vi "test_simple_examples with timeout.vi"() -> ()   [LabVIEW 2018, in "LV-0mq-Julia_roundtrip-lib.lvlib"]
uses:
  LV-0mq-Julia_roundtrip-lib.lvlib
  Server or client state.ctl
  detailed error info.ctl
  StackFrame.ctl
  simple examples functions.ctl
  ZMQ timeouts.ctl
  Commands.ctl
  commands LV2Jl.ctl
  482f2ec0-5302-44bb-bdd2-45c372870067.vi
  edf81fa3-46bf-427f-9605-85b461656974.vi
  d2cb43a9-9305-42fb-ad58-bce983510195.vi
  9182218e-1e17-4e73-8c4b-7de0f475a335.vi
  35a44a82-786b-41ea-be73-9a4468e4df9d.vi
  482f2ec0-5302-44bb-bdd2-45c372870067.vi/9ed5a05b-029a-4cf9-8f74-86d17c033540.vi
  482f2ec0-5302-44bb-bdd2-45c372870067.vi/431fdeb3-535d-48a6-80d3-ce07043e4822.vi
  482f2ec0-5302-44bb-bdd2-45c372870067.vi/6e3a5974-e93f-4958-8e58-bfe5222df237.vi
  edf81fa3-46bf-427f-9605-85b461656974.vi/dd2a08ad-0639-467b-9435-389f4bd48a85.vi
  d2cb43a9-9305-42fb-ad58-bce983510195.vi/e28c4e1c-617d-4a26-8291-f58a5accd33d.vi
  d2cb43a9-9305-42fb-ad58-bce983510195.vi/697b26af-9cff-4296-98ec-fa9d12ca8fdc.vi
  d2cb43a9-9305-42fb-ad58-bce983510195.vi/17159f77-75f5-4b7b-8d47-844af2eb1bcd.vi
  9182218e-1e17-4e73-8c4b-7de0f475a335.vi/6b7feeb5-19de-417f-bcbc-aec3b1e8345f.vi
  9182218e-1e17-4e73-8c4b-7de0f475a335.vi/7970c5bc-6f8c-498d-9eee-822ea5f26e23.vi
  9182218e-1e17-4e73-8c4b-7de0f475a335.vi/2f2cc08c-6f15-46a0-b24a-2c0737e5dd5e.vi
  35a44a82-786b-41ea-be73-9a4468e4df9d.vi/edd291af-888e-4547-8763-33a9db2b2a61.vi
  35a44a82-786b-41ea-be73-9a4468e4df9d.vi/9c0ac3f0-dad9-4795-8f5f-702d875dafaa.vi
  edf81fa3-46bf-427f-9605-85b461656974.vi/dd2a08ad-0639-467b-9435-389f4bd48a85.vi/1040e0bc-00ab-48b1-9004-b2897991f2c6.vi
  35a44a82-786b-41ea-be73-9a4468e4df9d.vi/edd291af-888e-4547-8763-33a9db2b2a61.vi/c75629c6-22a1-4cf2-848a-1de687213dd2.vi
  35a44a82-786b-41ea-be73-9a4468e4df9d.vi/edd291af-888e-4547-8763-33a9db2b2a61.vi/58d0dd4f-d013-483e-a73a-a72c22b2f5d6.vi
  edf81fa3-46bf-427f-9605-85b461656974.vi/dd2a08ad-0639-467b-9435-389f4bd48a85.vi/1040e0bc-00ab-48b1-9004-b2897991f2c6.vi/e9506487-c1a2-4aa8-b83c-f353e91e5b82.vi
  35a44a82-786b-41ea-be73-9a4468e4df9d.vi/edd291af-888e-4547-8763-33a9db2b2a61.vi/c75629c6-22a1-4cf2-848a-1de687213dd2.vi/f86c6b3b-20ab-4607-a249-4edff951d1c3.vi
  check ID validity.vi
  bindata_descr to JSON.vi
  check cluster field names.vi
  concat JSON.vi
  <vilib>/Utility/error.llb/Error Cluster From Error Code.vi
  <vilib>/measure/NI_MABase.lvlib
panel:
  out "fns":string[](array[string])
  out "ZMQ prev Timeouts out":T1={"SNDTIMEO"=-1, "RCVTIMEO"=-1}
  out "Jl Server state":T2
  in  "execution control pages":enum32{"Start", "go - test"}(tab)
  in  "go":bool caption="go (Julia Server started externally)"
  in  "Start with Julia":bool caption="Start Julia Server and go"
  in  "p":dbl=1.0
  in  "fn":T3 caption="select function at Server" items=["arr_amplitude", "arr_length", "arr_mean", "arr_median", "arr_rms", "vec_amplify", "vec_attenuate", "vec_power"]
  in  "trim_at_begin":dbl
  in  "trim_at_end":dbl
  in  "Group":T4(tab)
  out "Server response":dbl
  out "data received plot":dbl[](graph)
  out "data received":dbl[](array[numeric]) format="%.3f"
  out "RMS":dbl
  out "detailed error info":T5
  out "current error":errorcluster
  out "final error":errorcluster
  out "short err code":u8
  in  "tones":T7(array[cluster])=[{"frequency"=10.0, "amplitude"=1.0, "phase"=0.0}, {"frequency"=20.0, "amplitude"=0.1, "phase"=0.0}] {"phase" format="%.2p"; "amplitude" format="%0.2p"; "frequency" format="%0.2p"}
  in  "noise (rms)":dbl=0.1 format="%.2p"
  in  "offset":dbl format="%.2p"
  in  "sampling info":cluster{"Fs":dbl, "#s":dbl}={"Fs"=1000.0, "#s"=1000.0} {"Fs" format="%.2p"}
  in  "next":bool
  out "data sent to server":dbl[](graph)
  out "data sent":dbl[](array[numeric]) format="%.3f"
  out "function name":string
  in  "stop this VI only":bool
  in  "stop both this VI and Julia Server":bool
  # "generate sample array"
  # "function and parameter"
  # "enter a negative or a large positive value to cause an exception"
  # "data returned by server"
  # "data sent to server"
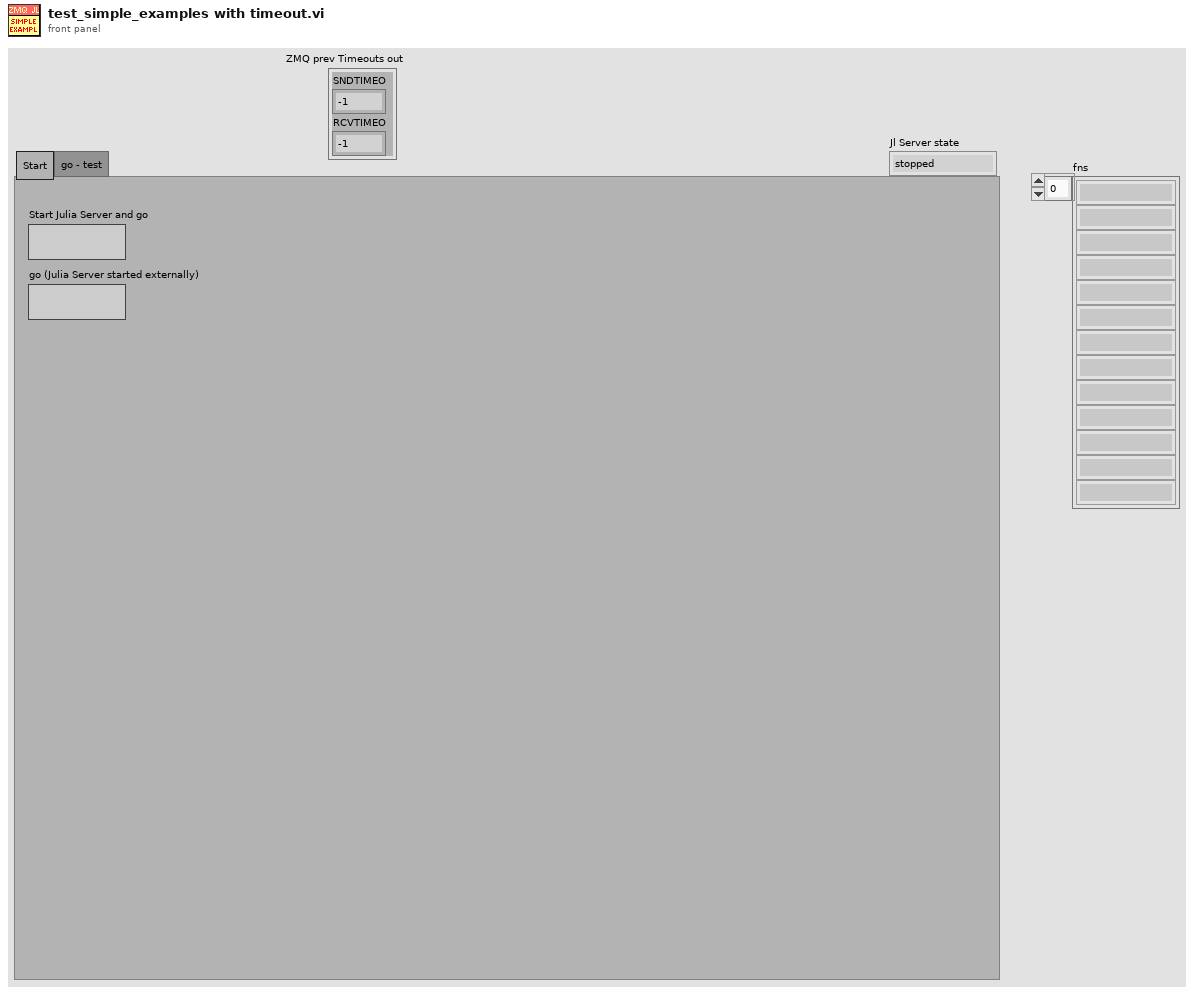
[diagram p1: front panel]
types:
  T1 = typedef "LV-0mq-Julia_roundtrip-lib.lvlib/ZMQ timeouts.ctl" = cluster{"SNDTIMEO":i32, "RCVTIMEO":i32}
  T2 = typedef "LV-0mq-Julia_roundtrip-lib.lvlib/Server or client state.ctl" = enum16{"stopped", "running", "unknown"}
  T3 = typedef "LV-0mq-Julia_roundtrip-lib.lvlib/simple examples functions.ctl" = u16
  T4 = enum32{"fns returning scalar", "fns returning vector", "error"}
  T5 = typedef "LV-0mq-Julia_roundtrip-lib.lvlib/detailed error info.ctl" = cluster{"exception_or_info":string, "trace":T6[]}
  T6 = typedef "LV-0mq-Julia_roundtrip-lib.lvlib/StackFrame.ctl" = cluster{"frame_summary":string, "func":string, "linfo":string, "file":string, "line":i32, "pointer":u64, "from_c":bool, "inlined":bool}
  T7 = cluster{"frequency":dbl, "amplitude":dbl, "phase":dbl}[]
  T8 = typedef "LV-0mq-Julia_roundtrip-lib.lvlib/commands LV2Jl.ctl" = u8
  T9 = typedef "LV-0mq-Julia_roundtrip-lib.lvlib/Commands.ctl" = enum16{"Start Jl-server & Init LV-client", "Send request & Get response ", "Stop Jl-server & Cleanup LV-client", "Cleanup LV-client", "Start Jl-server", "Stop Jl-server", "Init LV-Client", "Cleanup LV-Client", "(not allowed)", "Set LV Client state", "Set Jl Server state", "set ZMQ timeout", "read ZMQ timeout", "read-out state"}
  T10 = enum8{"Enabled", "Disabled", "Disabled and Grayed Out"}
  T11 = typedef "LV-0mq-Julia_roundtrip-lib.lvlib/Bindata&description.ctl" = cluster{"bindata_descr":T12[], "bindata":u8[]}
  T12 = typedef "LV-0mq-Julia_roundtrip-lib.lvlib/Bindata description.ctl" = cluster{"nofbytes":i32, "numtype":string, "start":i32, "arrdims":i32[], "kwarg_name":string, "category":string}
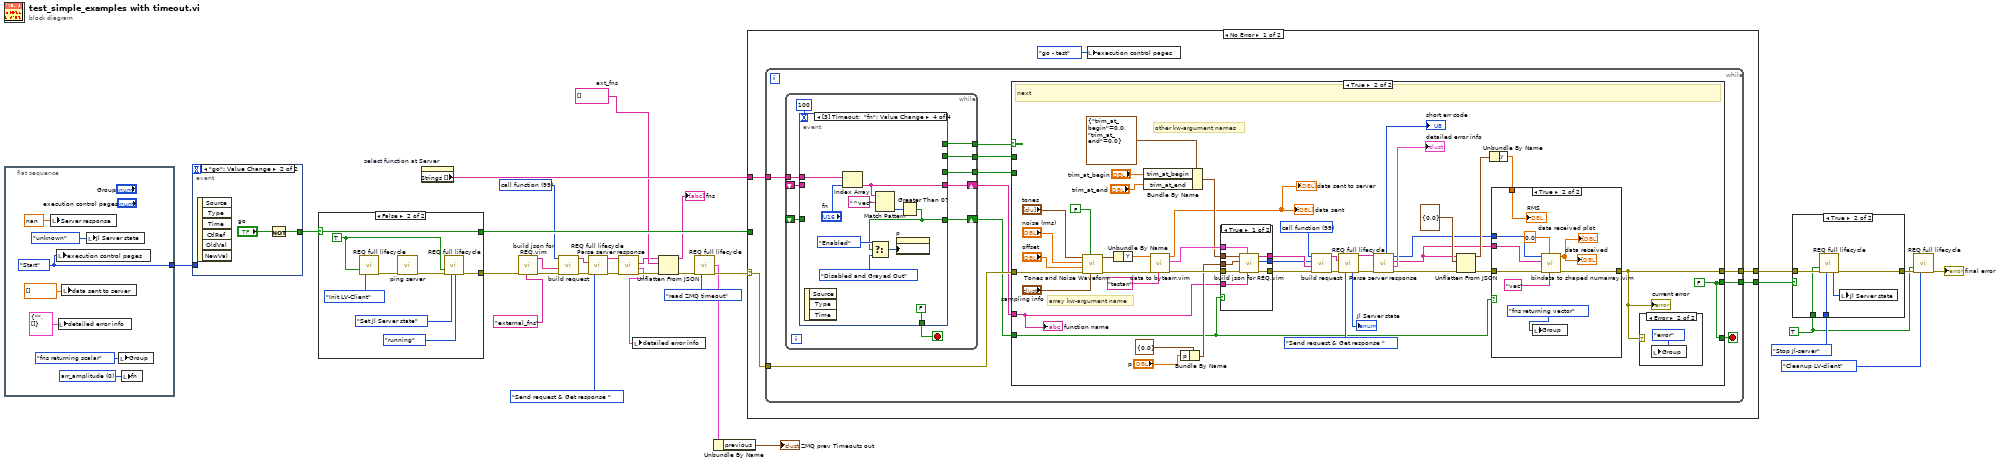
[diagram p0: block diagram]
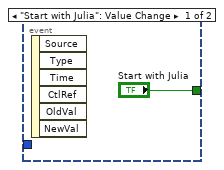
[diagram p2: hidden frame]
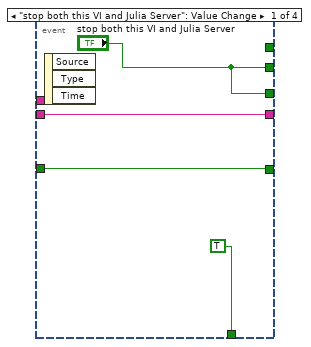
[diagram p3: hidden frame]
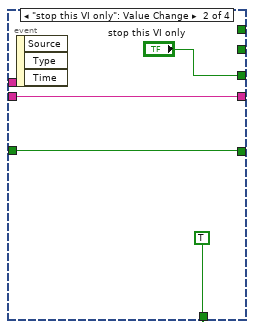
[diagram p4: hidden frame]
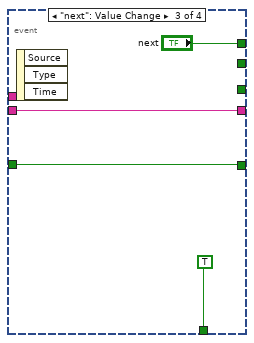
[diagram p5: hidden frame]
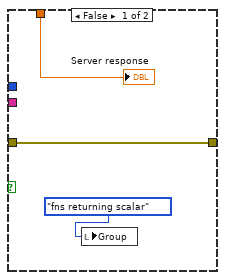
[diagram p7: hidden frame]
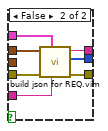
[diagram p8: hidden frame]
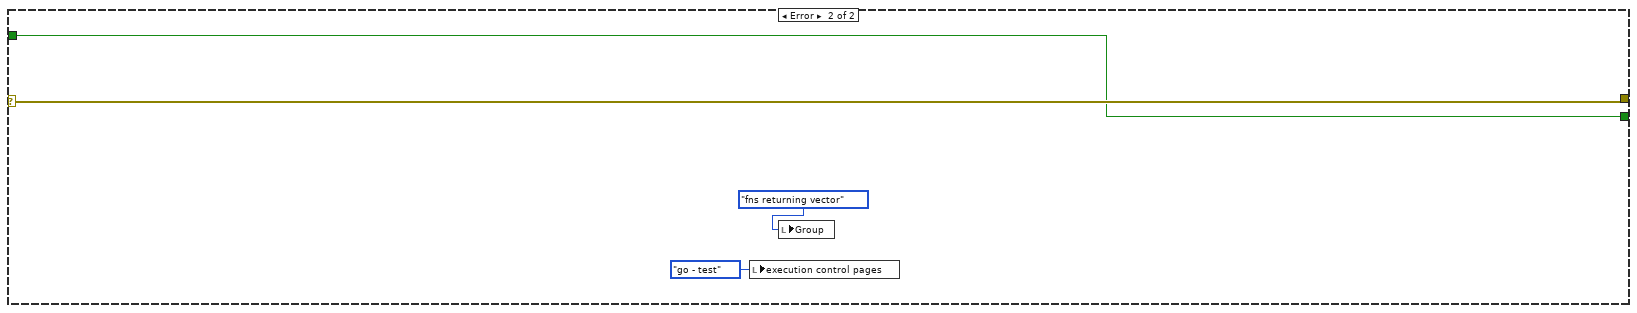
[diagram p10: hidden frame]
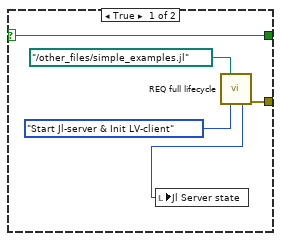
[diagram p11: hidden frame]
diagram:
  w4 = string[] []  # ext_fns
  w13 = T8 99 items=["call function"=99, "ping"=112, "stop"=115, "unused"=254] ("Command")
  w26 = TRUE ("Force command")
  n1 = flat-sequence {
    tunnel: [w38] -> w21
    frame #0 {
      w32 = T3 0 items=["arr_amplitude", "arr_length", "arr_mean", "arr_median", "arr_rms", "vec_amplify", "vec_attenuate", "vec_power"] ("fn")
      w38 = enum32{"Start", "go - test", "finish"}."Start" ("execution control pages")
      n2 = local write "Server response"(nan ("Server response")) -> ()
      n3 = local write "execution control pages"(w38) -> ()
      n4 = local write "detailed error info"(T5 {"exception_or_info"="", "trace"=[]} ("detailed error info")) -> ()
      n5 = local write "data sent to server"(dbl[] []) -> ()
      n6 = local write "Jl Server state"(Server_or_client_state."unknown" ("Jl Server state out")) -> ()
      n7 = local write "Group"(T4."fns returning scalar" ("Group")) -> ()
      n8 = local write "fn"(w32) -> ()
    }
  }
  n9 = event shown="[1] \"go\": Value Change" {
    selector: _ -> [_ _]
    dyn-events: _ -> [_ _]
    timeout: _ -> [_ _]
    tunnel: ["Start with Julia" w40] -> w24
    tunnel: w21 -> [_ _]
    event "Start with Julia": Value Change {
      n10 = event-data() -> ()  [unwired: 1 in, 6 out]
    }
    event "go": Value Change {
      n11 = event-data() -> ()  [unwired: 1 in, 6 out]
      n12 = Not(x="go") -> (.not. x?=w40:bool)
    }
  }
  n13 = case shown="False" w24 {
    selector: w24 -> [w43 w49]
    tunnel: [w45 w50] -> w12
    tunnel: [w43 w49] -> w22
    frame True {
      n14 = call "REQ full lifecycle.vi"("Julia user functions script"=path "../other_files/simple_examples.jl", "command"=Commands."Start Jl-server & Init LV-client") -> ("Jl Server state out"=w42:T2, "error out"=w45:errorcluster)  [unwired: 7 in, 5 out]
      n15 = local write "Jl Server state"(w42) -> ()
    }
    frame False {
      w52 = TRUE ("Force command")
      n16 = call "REQ full lifecycle.vi"("Force command"=w52, "command"=Commands."Init LV-Client") -> ("error out"=w48:errorcluster)  [unwired: 7 in, 6 out]
      n17 = call "ping server.vi"("error in"=w48) -> ("error out"=w47:errorcluster)  [unwired: 9 in, 1 out]
      n18 = call "REQ full lifecycle.vi"("Force command"=w52, "error in"=w47, "command"=Commands."Set Jl Server state", "Jl Server state in"=Server_or_client_state."running") -> ("error out"=w50:errorcluster)  [unwired: 5 in, 6 out]
    }
  }
  n19 = property on="select function at Server" class="Ring (strict)"() -> ("Strings []"=w23:string[])  [unwired: 2 in, 2 out]
  n20 = call "build json for REQ.vim"("fun2call"="external_fns", "error in (no error)"=w12) -> ("error out"=w11:errorcluster, "JSON string out"=w10:string)  [unwired: 7 in, 1 out]
  n21 = call "build request.vi"("error in (no error)"=w11, "JSON data"=w10, "Command"=w13) -> ("error out"=w15:errorcluster, "REQ string"=w14:string)  [unwired: 7 in]
  n22 = call "REQ full lifecycle.vi"("data to send"=w14, "error in"=w15, "command"=Commands."Send request & Get response ") -> ("server response"=w7:string, "error out"=w8:errorcluster)  [unwired: 6 in, 5 out]
  n23 = call "Parse server response.vi"("error in (no error)"=w8, "server response in"=w7) -> ("error out"=w6:errorcluster, "detailed error info"=w1:T5, "JSON out"=w3:string)  [unwired: 3 in, 4 out]
  n24 = local write "detailed error info"(w1) -> ()
  n25 = Unflatten From JSON(JSON string=w3, type and defaults=w4, error in (no error)=w6) -> (value=→"fns":string[], error out=w5:errorcluster)  [unwired: 4 in]
  n26 = call "REQ full lifecycle.vi"("error in"=w5, "command"=Commands."read ZMQ timeout") -> ("ZMQ timeouts out"=w18:cluster{"previous":T1, "current":T1}, "error out"=w20:errorcluster)  [unwired: 7 in, 5 out]
  n27 = Unbundle By Name(w18) -> ("previous"=→"ZMQ prev Timeouts out":T1)
  n28 = case shown="No Error" w20 {
    selector: w20 -> [w58 w179]
    tunnel: [w59 w179] -> w31
    tunnel: [w57 w178] -> w25
    tunnel: w23 -> [w56 _]
    tunnel: w22 -> [_ w178]
    frame No Error {
      n29 = while {
        tunnel: w58 -> [w68]
        tunnel: [w69] -> w59
        tunnel: [w65] -> w57
        tunnel: w56 -> [w63]
        stop <- w66 stop-if-true
        n30 = while {
          tunnel: [w79] -> w67
          tunnel: [w78] -> w64
          tunnel: w63 -> [w75]
          shift-right: [w74] -> w62
          shift-left: _ -> [w71]
          shift-right: [w73] -> w61
          shift-left: _ -> [w72]
          tunnel: [w70] -> w60
          stop <- w77 stop-if-true
          n31 = event shown="[3] Timeout;  \"fn\": Value Change" {
            selector: _ -> [_ _ _ _]
            dyn-events: _ -> [_ _ _ _]
            timeout: 100 -> [_ _ _ _]
            tunnel: ["stop both this VI and Julia Server" _ _ _] -> w78
            tunnel: [_ _ "next" _] -> w79
            tunnel: [TRUE TRUE TRUE FALSE] -> w77
            tunnel: w75 -> [_ _ _ w95]
            tunnel: [w81 w85 w89 w94] -> w74
            tunnel: [w82 w86 w88 w93] -> w73
            tunnel: w72 -> [w82 w86 w88 _]
            tunnel: w71 -> [w81 w85 w89 _]
            tunnel: ["stop both this VI and Julia Server" "stop this VI only" _ _] -> w70
            event "stop both this VI and Julia Server": Value Change {
              n32 = event-data() -> ()  [unwired: 1 in, 3 out]
            }
            event "stop this VI only": Value Change {
              n33 = event-data() -> ()  [unwired: 1 in, 3 out]
            }
            event "next": Value Change {
              n34 = event-data() -> ()  [unwired: 1 in, 3 out]
            }
            event Timeout; Value Change {
              n35 = event-data() -> ()  [unwired: 1 in, 3 out]
              n36 = Index Array(array=w95, index="fn") -> (element=w93:string)
              n37 = Match Pattern(string=w93, regular expression="^vec") -> (offset past match=w99:i32)  [unwired: 1 in, 3 out]
              n38 = Greater Than 0?(x=w99) -> (x > 0?=w94:bool)
              n39 = Select(t=T10."Enabled" ("Disabled"), s=w94, f=T10."Disabled and Grayed Out" ("Disabled")) -> (s? t:f=w101:T10)
              n40 = property on="p" class="DigNum (strict)"("DisabledEnum"=w101) -> ()  [unwired: 2 in, 2 out]
            }
          }
        }
        n41 = case shown="True" w67 {
          tunnel: [w104 w111] -> w69
          tunnel: w68 -> [w104 w118]
          tunnel: [w103 w116] -> w66
          tunnel: w60 -> [w103 _]
          tunnel: [w102 w116] -> w65
          tunnel: w64 -> [w102 _]
          tunnel: w62 -> [_ w107]
          tunnel: w61 -> [_ w106]
          frame False {
            # "stop"
          }
          frame True {
            w116 = FALSE ("stop this VI only")
            w141 = T8 99 items=["call function"=99, "ping"=112, "stop"=115] ("Command")
            # "other kw-argument names"
            # "array kw-argument name"
            # "next"
            n42 = call <vilib>:"Tones and Noise Waveform.vi"("sampling info"="sampling info", "reset signal"=FALSE, "error in (no error)"=w118, "offset"="offset", "noise (rms)"="noise (rms)", "tones"="tones") -> ("error out"=w119:errorcluster, "signal out"=w125:waveform(dbl))  [unwired: 4 in]
            n43 = Unbundle By Name(w125) -> ("Y"=w120:dbl[])
            n44 = Bundle By Name(cluster=cluster{"trim_at_begin":dbl, "trim_at_end":dbl} {"trim_at_begin"=0.0, "trim_at_end"=0.0}, "trim_at_begin"="trim_at_begin", "trim_at_end"="trim_at_end") -> (w129:cluster{"trim_at_begin":dbl, "trim_at_end":dbl})
            n45 = call "data to bytearr.vim"("kwarg_name"="testarr", "error in (no error)"=w119, "data in"=w120) -> ("error out"=w132:errorcluster, "Bindata & descr out"=w133:T11, "flattened data out"=→"data sent" →"data sent to server":dbl[])  [unwired: 6 in]
            n46 = Bundle By Name(cluster=cluster{"p":dbl} {"p"=0.0}, "p"="p") -> (w115:cluster{"p":dbl})
            n47 = case shown="True" w107 {
              tunnel: [w167 w174] -> w146
              tunnel: [w166 w173] -> w138
              tunnel: [w165 w172] -> w137
              tunnel: w133 -> [w164 w171]
              tunnel: w132 -> [w163 w170]
              tunnel: w129 -> [w162 w169]
              tunnel: w106 -> [w161 w168]
              tunnel: w115 -> [w160 _]
              frame True {
                n48 = call "build json for REQ.vim"("fun2call"=w161, "Bindata & descr in"=w164, "error in (no error)"=w163, "Arguments 2"=w160, "Arguments 1"=w162) -> ("error out"=w167:errorcluster, "bindata out"=w165:u8[], "JSON string out"=w166:string)  [unwired: 4 in]
              }
              frame False {
                n49 = call "build json for REQ.vim"("fun2call"=w168, "Bindata & descr in"=w171, "error in (no error)"=w170, "Arguments 1"=w169) -> ("error out"=w174:errorcluster, "bindata out"=w172:u8[], "JSON string out"=w173:string)  [unwired: 5 in]
              }
            }
            n50 = call "build request.vi"("error in (no error)"=w146, "JSON data"=w138, "binary data"=w137, "Command"=w141) -> ("error out"=w144:errorcluster, "REQ string"=w145:string)  [unwired: 6 in]
            n51 = call "REQ full lifecycle.vi"("data to send"=w145, "error in"=w144, "command"=Commands."Send request & Get response ") -> ("server response"=w105:string, "Jl Server state out"=→"Jl Server state":T2, "error out"=w143:errorcluster)  [unwired: 6 in, 4 out]
            n52 = call "Parse server response.vi"("error in (no error)"=w143, "server response in"=w105) -> ("error out"=w136:errorcluster, "detailed error info"=→"detailed error info":T5, "JSON out"=w109:string, "binary data"=w110:u8[], "return code"=→"short err code":u8)  [unwired: 3 in, 2 out]
            n53 = Unflatten From JSON(JSON string=w109, type and defaults=cluster{"y":dbl} {"y"=0.0} ("parsed response"), error in (no error)=w136) -> (value=w134:cluster{"y":dbl}, error out=w112:errorcluster)  [unwired: 4 in]
            n54 = Unbundle By Name(w134) -> ("y"=w108:dbl)
            n55 = case shown="True" w107 {
              tunnel: w112 -> [w150 w158]
              tunnel: [w150 w157] -> w111
              tunnel: w110 -> [_ w156]
              tunnel: w109 -> [_ w155]
              tunnel: w108 -> [w148 w152]
              frame False {
                n56 = local write "Group"(T4."fns returning scalar" ("Group")) -> ()
                "Server response" <- w148
              }
              frame True {
                n57 = local write "Group"(T4."fns returning vector" ("Group")) -> ()
                n58 = call "bindata to shaped numarray.vim"("kwarg_name"="vec", "data type"=0.0, "error in (no error)"=w158, "bindata_descr"=w155, "binary data"=w156) -> ("error out"=w157:errorcluster, "numarray 1D"=→"data received plot" →"data received":dbl[])  [unwired: 3 in, 2 out]
                "RMS" <- w152
              }
            }
            "current error" <- w111
            n59 = case shown="Error" w111 {
              frame No Error {
              }
              frame Error {
                n60 = local write "Group"(T4."error" ("Group")) -> ()
              }
            }
            "function name" <- w106
          }
        }
      }
      n61 = local write "execution control pages"(enum32{"Start", "go - test", "finish"}."go - test" ("execution control pages")) -> ()
    }
    frame Error {
      n62 = local write "execution control pages"(enum32{"Start", "go - test", "finish"}."go - test" ("execution control pages")) -> ()
      n63 = local write "Group"(T4."fns returning vector" ("Group")) -> ()
    }
  }
  n64 = case shown="True" w25 {
    tunnel: w31 -> [w180 w185]
    tunnel: Commands."Stop Jl-server" ("command") -> [_ w184]
    tunnel: [w180 w183] -> w29
    tunnel: w26 -> [_ w182]
    frame False {
    }
    frame True {
      n65 = call "REQ full lifecycle.vi"("Force command"=w182, "error in"=w185, "command"=w184) -> ("Jl Server state out"=w181:T2, "error out"=w183:errorcluster)  [unwired: 6 in, 5 out]
      n66 = local write "Jl Server state"(w181) -> ()
    }
  }
  n67 = call "REQ full lifecycle.vi"("Force command"=w26, "error in"=w29, "command"=Commands."Cleanup LV-client") -> ("error out"=→"final error":errorcluster)  [unwired: 6 in, 6 out]
